vi "CameraConfig.vi"(11 "IO Cluster In":T1={"Error"={"status"=FALSE, "code"=0, "source"=""}, "Encoder Calibration Values"=[22, 216], "Update Calibration"=FALSE, "JPEG Resolutions"=3, "Raw Resolutions"=1, "Image Mode"=enum."RAW Gray Scale", "FPGA Ref"=refnum} {"JPEG Resolutions" items=["160x128"=3, "320x240"=5, "640x480"=7]; "Raw Resolutions" items=["80x60"=1, "160x120"=3, "128x128"=9, "128x96"=11]}) -> (1 "Configuration Complete":bool, 3 "IO Cluster Out":T1={"Error"={"status"=FALSE, "code"=0, "source"=""}, "Encoder Calibration Values"=[22, 216], "Update Calibration"=FALSE, "JPEG Resolutions"=3, "Raw Resolutions"=1, "Image Mode"=enum."RAW Gray Scale", "FPGA Ref"=refnum} {"JPEG Resolutions" items=["160x128"=3, "320x240"=5, "640x480"=7]; "Raw Resolutions" items=["80x60"=1, "160x120"=3, "128x128"=9, "128x96"=11]}, 6 "Image Mode Set":bool)   [LabVIEW 2019]
uses:
  QNET MS IO Cluster.ctl
  <vilib>/Utility/error.llb/Error Cluster From Error Code.vi
  <vilib>/rvi/errors/niLvFpgaAdjustHostInterfaceError.vi
  <vilib>/rvi/interface/nirviReadWriteControl/nirviReadWriteControl.xnode
  NiFpgaLv.dll
  <vilib>/rvi/interface/Simulation/niFpgaSimulationCallBeginRW.vi
panel:
  out "Baud Set":bool
  out "byte array":u8[](array[numeric]) format="%02x"
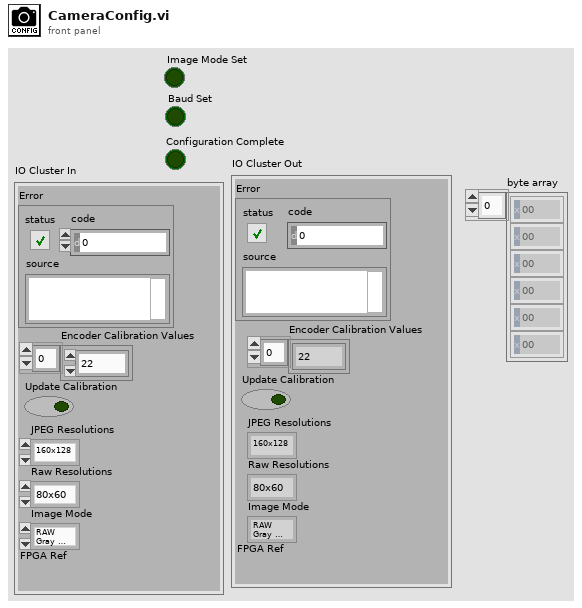
[diagram p1: front panel]
types:
  T1 = typedef "QNET MS IO Cluster.ctl" = cluster{"Error":errorcluster, "Encoder Calibration Values":i32[], "Update Calibration":bool, "JPEG Resolutions":u16, "Raw Resolutions":u16, "Image Mode":enum16{"RAW RGB", "RAW Gray Scale", "JPEG"}, "FPGA Ref":refnum<k20>}
  T2 = enum16{"Config Image Mode", "Image Mode ACK", "Config Baud", "Baud ACK", "Error"}
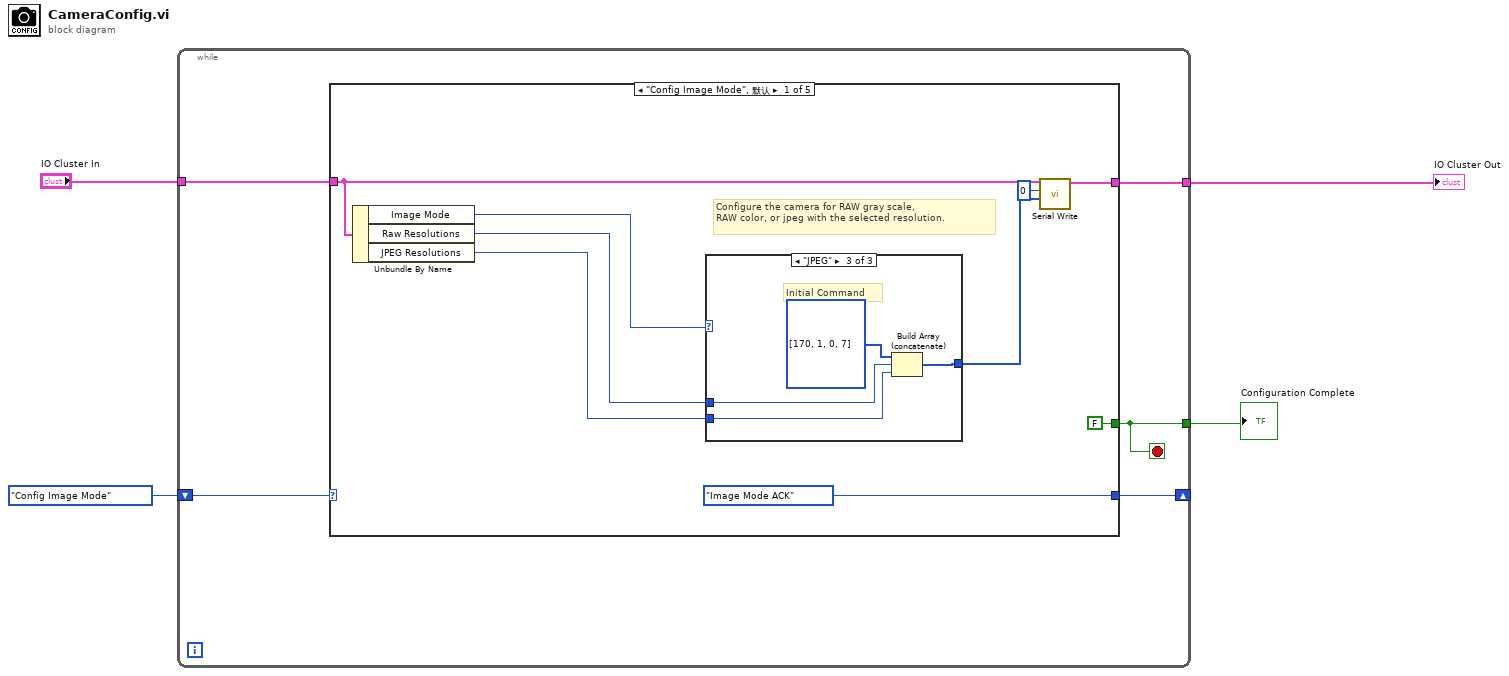
[diagram p0: block diagram]
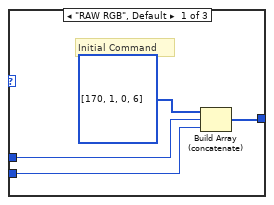
[diagram p2: hidden frame]
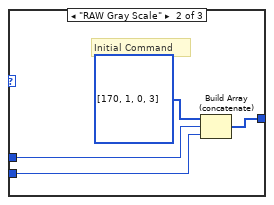
[diagram p3: hidden frame]
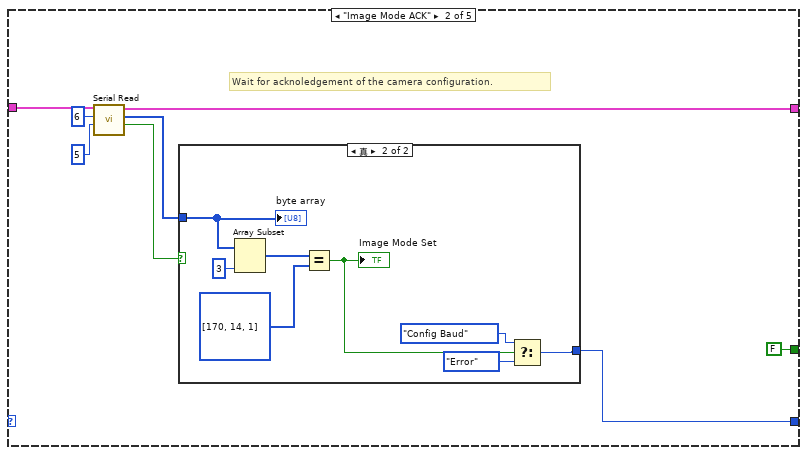
[diagram p4: hidden frame]
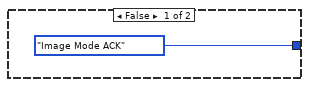
[diagram p5: hidden frame]
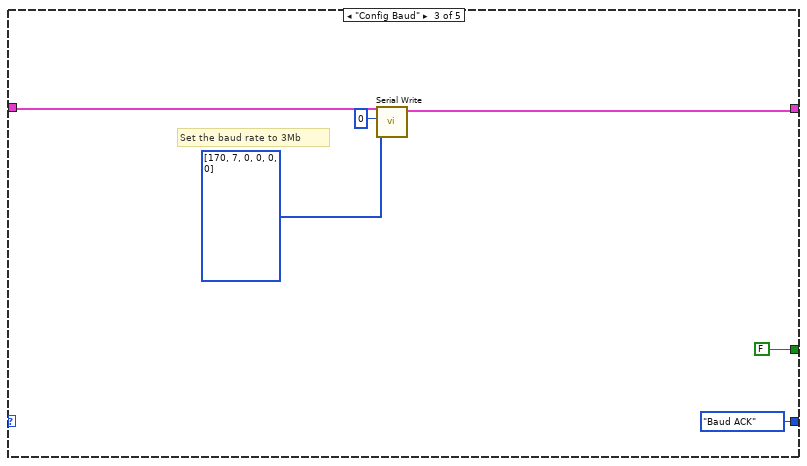
[diagram p6: hidden frame]
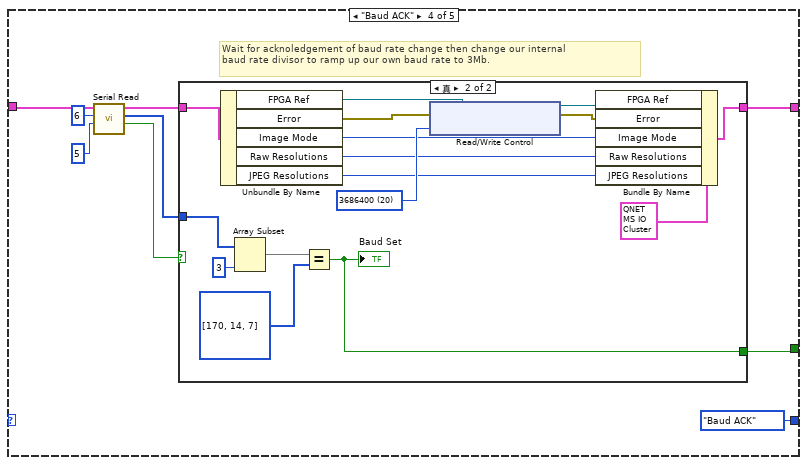
[diagram p7: hidden frame]
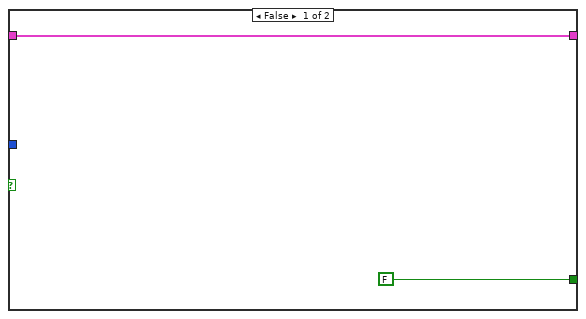
[diagram p8: hidden frame]
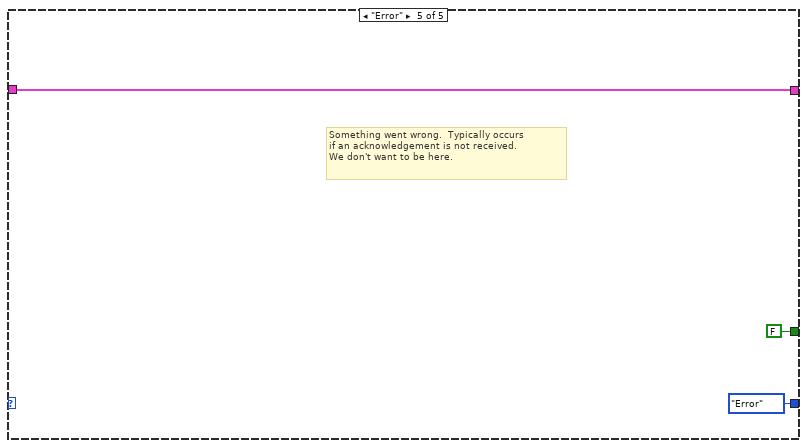
[diagram p9: hidden frame]
diagram:
  n1 = while {
    tunnel: [w9] -> w4
    shift-right: [w8] -> _
    shift-left: T2."Config Image Mode" -> [w7]
    tunnel: "IO Cluster In" -> [w6]
    tunnel: [w5] -> w1
    stop <- w9 stop-if-true
    n2 = case shown="\"Config Image Mode\", 默认" w7 {
      tunnel: [T2."Image Mode ACK" w34 T2."Baud ACK" ("f") T2."Baud ACK" ("f") T2."Error" ("f")] -> w8
      tunnel: [FALSE FALSE FALSE w57 FALSE] -> w9
      tunnel: w6 -> [w11 w32 w49 w55 w81]
      tunnel: [w10 w31 w48 w54 w81] -> w5
      frame "Config Image Mode", Default {
        # "Configure the camera for RAW gray scale,\nRAW color, or jpeg with the selected resolution."
        n3 = Unbundle By Name(w11) -> ("Image Mode"=w14:enum16{"RAW RGB", "RAW Gray Scale", "JPEG"}, "Raw Resolutions"=w13:u16, "JPEG Resolutions"=w12:u16)
        n4 = case shown="\"JPEG\"" w14 {
          tunnel: [w21 w25 w30] -> w18
          tunnel: w13 -> [w20 w24 w28]
          tunnel: w12 -> [w19 w23 w27]
          frame "RAW RGB", Default {
            # "Initial Command"
            n5 = Build Array (concatenate)(u8[] [170, 1, 0, 6], w20, w19) -> (w21:u16[])
          }
          frame "RAW Gray Scale" {
            # "Initial Command"
            n6 = Build Array (concatenate)(u8[] [170, 1, 0, 3], w24, w23) -> (w25:u16[])
          }
          frame "JPEG" {
            # "Initial Command"
            n7 = Build Array (concatenate)(u8[] [170, 1, 0, 7], w28, w27) -> (w30:u16[])
          }
        }
        n8 = call "Serial Write.vi"("Array"=w18, "Timeout (ms)"=0, "IO Cluster In"=w11) -> ("IO Cluster Out"=w10:T1)  [unwired: 8 in]
      }
      frame "Image Mode ACK" {
        # "Wait for acknoledgement of the camera configuration."
        n9 = call "Serial Read.vi"("Timeout (ms)"=5, "Number of Bytes to Read"=u32 6, "IO Cluster In"=w32) -> ("Data Valid"=w36:bool, "Data"=w35:u8[], "IO Cluster Out"=w31:T1)  [unwired: 4 in, 2 out]
        n10 = case shown="真" w36 {
          tunnel: w35 -> [_ w47]
          tunnel: [T2."Image Mode ACK" w41] -> w34
          frame False {
          }
          frame True {
            n11 = Array Subset(array=w47, length=3) -> (w45:u8[])  [unwired: 1 in]
            n12 = Equal?(x=w45, y=u8[] [170, 14, 1]) -> (x = y?=w43:bool)
            "Image Mode Set" <- w43
            n13 = Select(t=T2."Config Baud", s=w43, f=T2."Error") -> (s? t:f=w41:T2)
            "byte array" <- w47
          }
        }
      }
      frame "Config Baud" {
        # "Set the baud rate to 3Mb"
        n14 = call "Serial Write.vi"("Array"=u8[] [170, 7, 0, 0, 0, 0], "Timeout (ms)"=0, "IO Cluster In"=w49) -> ("IO Cluster Out"=w48:T1)  [unwired: 8 in]
      }
      frame "Baud ACK" {
        # "Wait for acknoledgement of baud rate change then change our internal\nbaud rate divisor to ramp up our own baud rate to 3Mb."
        n15 = call "Serial Read.vi"("Timeout (ms)"=5, "Number of Bytes to Read"=u32 6, "IO Cluster In"=w55) -> ("Data Valid"=w60:bool, "Data"=w59:u8[], "IO Cluster Out"=w56:T1)  [unwired: 4 in, 2 out]
        n16 = case shown="真" w60 {
          tunnel: w59 -> [_ w80]
          tunnel: [FALSE w76] -> w57
          tunnel: w56 -> [w63 w72]
          tunnel: [w63 w68] -> w54
          frame False {
          }
          frame True {
            w75 = u16 20 items=["9600"=8063, "19200"=4031, "38400"=2015, "57600"=1343, "115200"=671, "153600"=503, "230400"=335, "460800"=167, "921600"=83, "1228800"=62, "1843200"=41, "3686400"=20] ("Baud Rate")
            n17 = Unbundle By Name(w72) -> ("FPGA Ref"=w71:refnum<k20>, "Error"=w70:errorcluster, "Image Mode"=w69:enum16{"RAW RGB", "RAW Gray Scale", "JPEG"}, "Raw Resolutions"=w67:u16, "JPEG Resolutions"=w66:u16)
            n18 = Array Subset(array=w80, length=3) -> (w78:u8[])  [unwired: 1 in]
            n19 = Equal?(x=w78, y=u8[] [170, 14, 7]) -> (x = y?=w76:bool)
            "Baud Set" <- w76
            n20 = xnode "Read/Write Control"("FPGA VI引用输入"=w71, "错误输入"=w70, "UART Clock Divisor"=w75) -> ("FPGA VI引用输出"=w74:refnum<k20>, "错误输出"=w73:errorcluster)
            n21 = Bundle By Name(cluster=T1 {"Error"={"status"=FALSE, "code"=0, "source"=""}, "Encoder Calibration Values"=[22, 216], "Update Calibration"=FALSE, "JPEG Resolutions"=3, "Raw Resolutions"=1, "Image Mode"=enum."RAW Gray Scale", "FPGA Ref"=refnum} ("IO Cluster"), "FPGA Ref"=w74, "Error"=w73, "Image Mode"=w69, "Raw Resolutions"=w67, "JPEG Resolutions"=w66) -> (w68:T1)
          }
        }
      }
      frame "Error" {
        # "Something went wrong.  Typically occurs\nif an acknowledgement is not received.\nWe don't want to be here."
      }
    }
  }
  "Configuration Complete" <- w4
  "IO Cluster Out" <- w1
